vi "play-general-scan-with-autoID.vi"() -> ()   [LabVIEW 2017]
uses:
  <vilib>/addons/Control Design/_Model Construction/Model Typedefs.llb/CD State Space Model (MIMO).ctl
  <vilib>/addons/Control Design/_Model Construction/Model Typedefs.llb/CD General Elements.ctl
  fpga_VIs/fpga_subVIs_ssxy/fixed-point-ss/typeDefs/FXPControlParams-ss-xy.ctl
  controls/z-axis-params_v4_prescan.ctl
  controls/TF-params.ctl
  controls/scan_input_meta_data.ctl
  controls/scan-mode-CTL.ctl
  fpga_VIs/controls/supervisor-params.ctl
  fpga_VIs/controls/fpga-scan-status.ctl
  controls/boolean_info.ctl
  controls/auto_id_result.ctl
  subVIs/auto-sys-id/controls/SOS_frf_data.ctl
  fpga_interface_lib/fpga_interface_types/cs-scan-inputs-TYPE.ctl
  <vilib>/userdefined/High Color/nirio_resource_hc.ctl
  controls/rasterMetaData_asCS.ctl
  <vilib>/FPGAPlugInAG/cRIO-9082/niLvFpga_Open_cRIO-9082.vi
  <vilib>/rvi/interface/common/dynamic/niFpgaDynamicAddResources.vi
  <vilib>/FPGAPlugInAG/Dynamic/niLvFpga_Reset_Dynamic.vi
  <vilib>/Utility/error.llb/Error Cluster From Error Code.vi
  <vilib>/rvi/errors/niLvFpgaAdjustHostInterfaceError.vi
  <vilib>/FPGAPlugInAG/Dynamic/niLvFpga_Run_Dynamic.vi
  fpga_interface_lib/acquire_FXP_16-5_FIFO_2.vi
  <vilib>/RVI Host/nirviSupport.llb/nirviErrorClusterFromErrorCode.vi
  <vilib>/FPGAPlugInAG/Dynamic/niLvFpga_Close_Dynamic.vi
  <vilib>/rvi/interface/nirviOpenFPGA/nirviOpenFPGA.xnode
  FPGA Bitfiles/afmimagingcontro_FPGATargetSPARTA_cs-scanningv5ssx.lvbitx
  <vilib>/rvi/interface/nirviMethod/nirviMethod.xnode
  <vilib>/rvi/interface/nirviReadWriteControl/nirviReadWriteControl.xnode
  <vilib>/rvi/interface/nirviCloseFPGA/nirviCloseFPGA.xnode
  <vilib>/rvi/interface/Simulation/niFpgaSimulationCallBeginRW.vi
  NiFpgaLv.dll
  fpga_interface_lib/fpga_interface.lvlib
  <vilib>/addons/_JKI.lib/Serialization/JSON/JKI JSON Serialization.lvlib
  <vilib>/rvi/interface/nirviMethod/StockFPGA_InlinedMethodWaitForSingleIRQ.vi
  <vilib>/FPGAPlugInAG/Dynamic/niLvFpga_WaitOnIrq_Dynamic.vi
  <vilib>/FPGAPlugInAG/Dynamic/niLvFpga_AcknowledgeIrq_Dynamic.vi
  <vilib>/addons/Control Design/_Model Construction/NI_LinSys_Model Typedefs.lvlib
panel:
  out "Array 3":T1(array[cluster])
  out "current-acquisition":i32
  out "state0-count":u64
  out "output cluster":T2={"xy_settled_samples_threshold"=15, "xy_error_threshold"=0.01, "zup_err_threshold"=0.10000228881835938, "prescan_samples"=5000, "TOL"=0.3, "collect_all"=TRUE, "numEntities"=0} {"TOL" format="%#_13g"}
  out "current-state":u8
  in  "Alert-on-Finish":bool
  out "state times":dbl[](array[numeric])
  out "ControlMatrices":T3
  in  "Tab Control":T4(tab)
  in  "Array 4":path[](array[path])
  in  "z_axis_params":T5={"z_u_max"=2.0, "setpoint_scan"=-0.3000030517578125, "Ki_scan"=0.07, "uz_safe"=0.2998046875, "Kiz_down"=0.045, "setpoint_up"=-0.8000030517578125, "do_Dz"=TRUE, "PID_while_xy_move"=FALSE, "TF_params"={"TF_order"=2, "Num"=[1.0, -1.9962076, 0.9990926, 0.0, 0.0, 0.0, 0.0, 0.0, 0.0], "Den"=[1.0, -1.9961313, 0.9990842, 0.0, 0.0, 0.0, 0.0, 0.0, 0.0]}, "KI_slope"=1.0, "enable_KI_sched"=FALSE, "KI_min"=0.0099945068359375, "KI_max"=0.1999969482421875} {"Kiz_down" format="%#_13g"; "Ki_scan" min=0 max=0.4 step=0.0025; "z_u_max" format="%#_13g"}
  in  "overwrite":bool
  in  "note-blob":string
  in  "state-machine-params":T2={"xy_settled_samples_threshold"=20, "xy_error_threshold"=0.01, "zup_err_threshold"=0.05100059509277344, "prescan_samples"=0, "TOL"=0.0259, "collect_all"=TRUE, "numEntities"=0} {"TOL" format="%#_13g"}
  in  "trigger-0":bool
  in  "STOP":bool
  out "CS Time":dbl
  in  "collect-0":bool
  in  "Continue":bool
  out "output-data-paths":path[](array[path])
  in  "file path (use dialog)":path=path "C:/Users/arnold/Documents/afm-cs/labview/first_res_fit-5-9-2019-sicon.json"
  in  "xy-gain-mult":dbl=1.0 min=0.0 max=1.0 step=1.0 format="%#_13g"
  in  "Load-Dinv":bool=TRUE
  in  "Swept-Sines-Control-Settings":cluster{"u-max":sgl, "offset":sgl, "Ki":sgl}={"u-max"=1.0, "offset"=0.1, "Ki"=0.0}
  in  "SS-amp":dbl=0.12 format="%#_13g"
  out "Bode amplitude":cluster{"W":dbl[], "Magnitude":dbl[]}[](graph) caption="Magnitude Graph"
  out "Channel 1":cluster{"W":dbl[], "Magnitude":dbl[]}[](graph) caption="Magnitude Graph"
  out "value":T7
  in  "Abort-swept-sines":bool
  in  "control_data_path":path=path "Z:/afm-cs/step-exps/LinControls-choose-zeta_5micron.json"
  in  "umax-xy":dbl=5.0 format="%#_13g"
  out "Gdrift-inv-xdir":T9 {"Transport Delay" format="%.2f"; "D" format="%#.5g"; "C" format="%#.5g"; "B" format="%#.5g"; "A" format="%#.5g"; "properties"."Sampling Time" format="%#.6p"; "properties"."Output Delays" format="%.4f"; "properties"."Input Delays" format="%.4f"}
  out "ControlParamsLin-ss":T11={"umax"=3.0, "Ns_obs/cntrl"=0, "ref_f_VEC"=[0.0, 0.0], "du_max"=0.0, "Nbar"=0.0, "Nhyst"=0, "Nsat"=0, "Ndrift+1"=0, "Ki-y"=0.01}
  in  "Ki-y":sgl=0.01
  out "scan-status":T12
  out "error out 2":errorcluster
  out "scan_meta":T14
  out "Kiscan-effective":dbl
  out "Kidown-effective":dbl
  out "K":dbl
  out "error out":errorcluster
  out "output-meta-data-path":path
  # "C:\\Users\\arnold\\Documents\\afm-cs\\labview\\first_res_fit-4-19-2019-sicon.json"
  # "make this come from input csv!"
  # "For the y-axis only, shouldnt ever really\nneed to change"
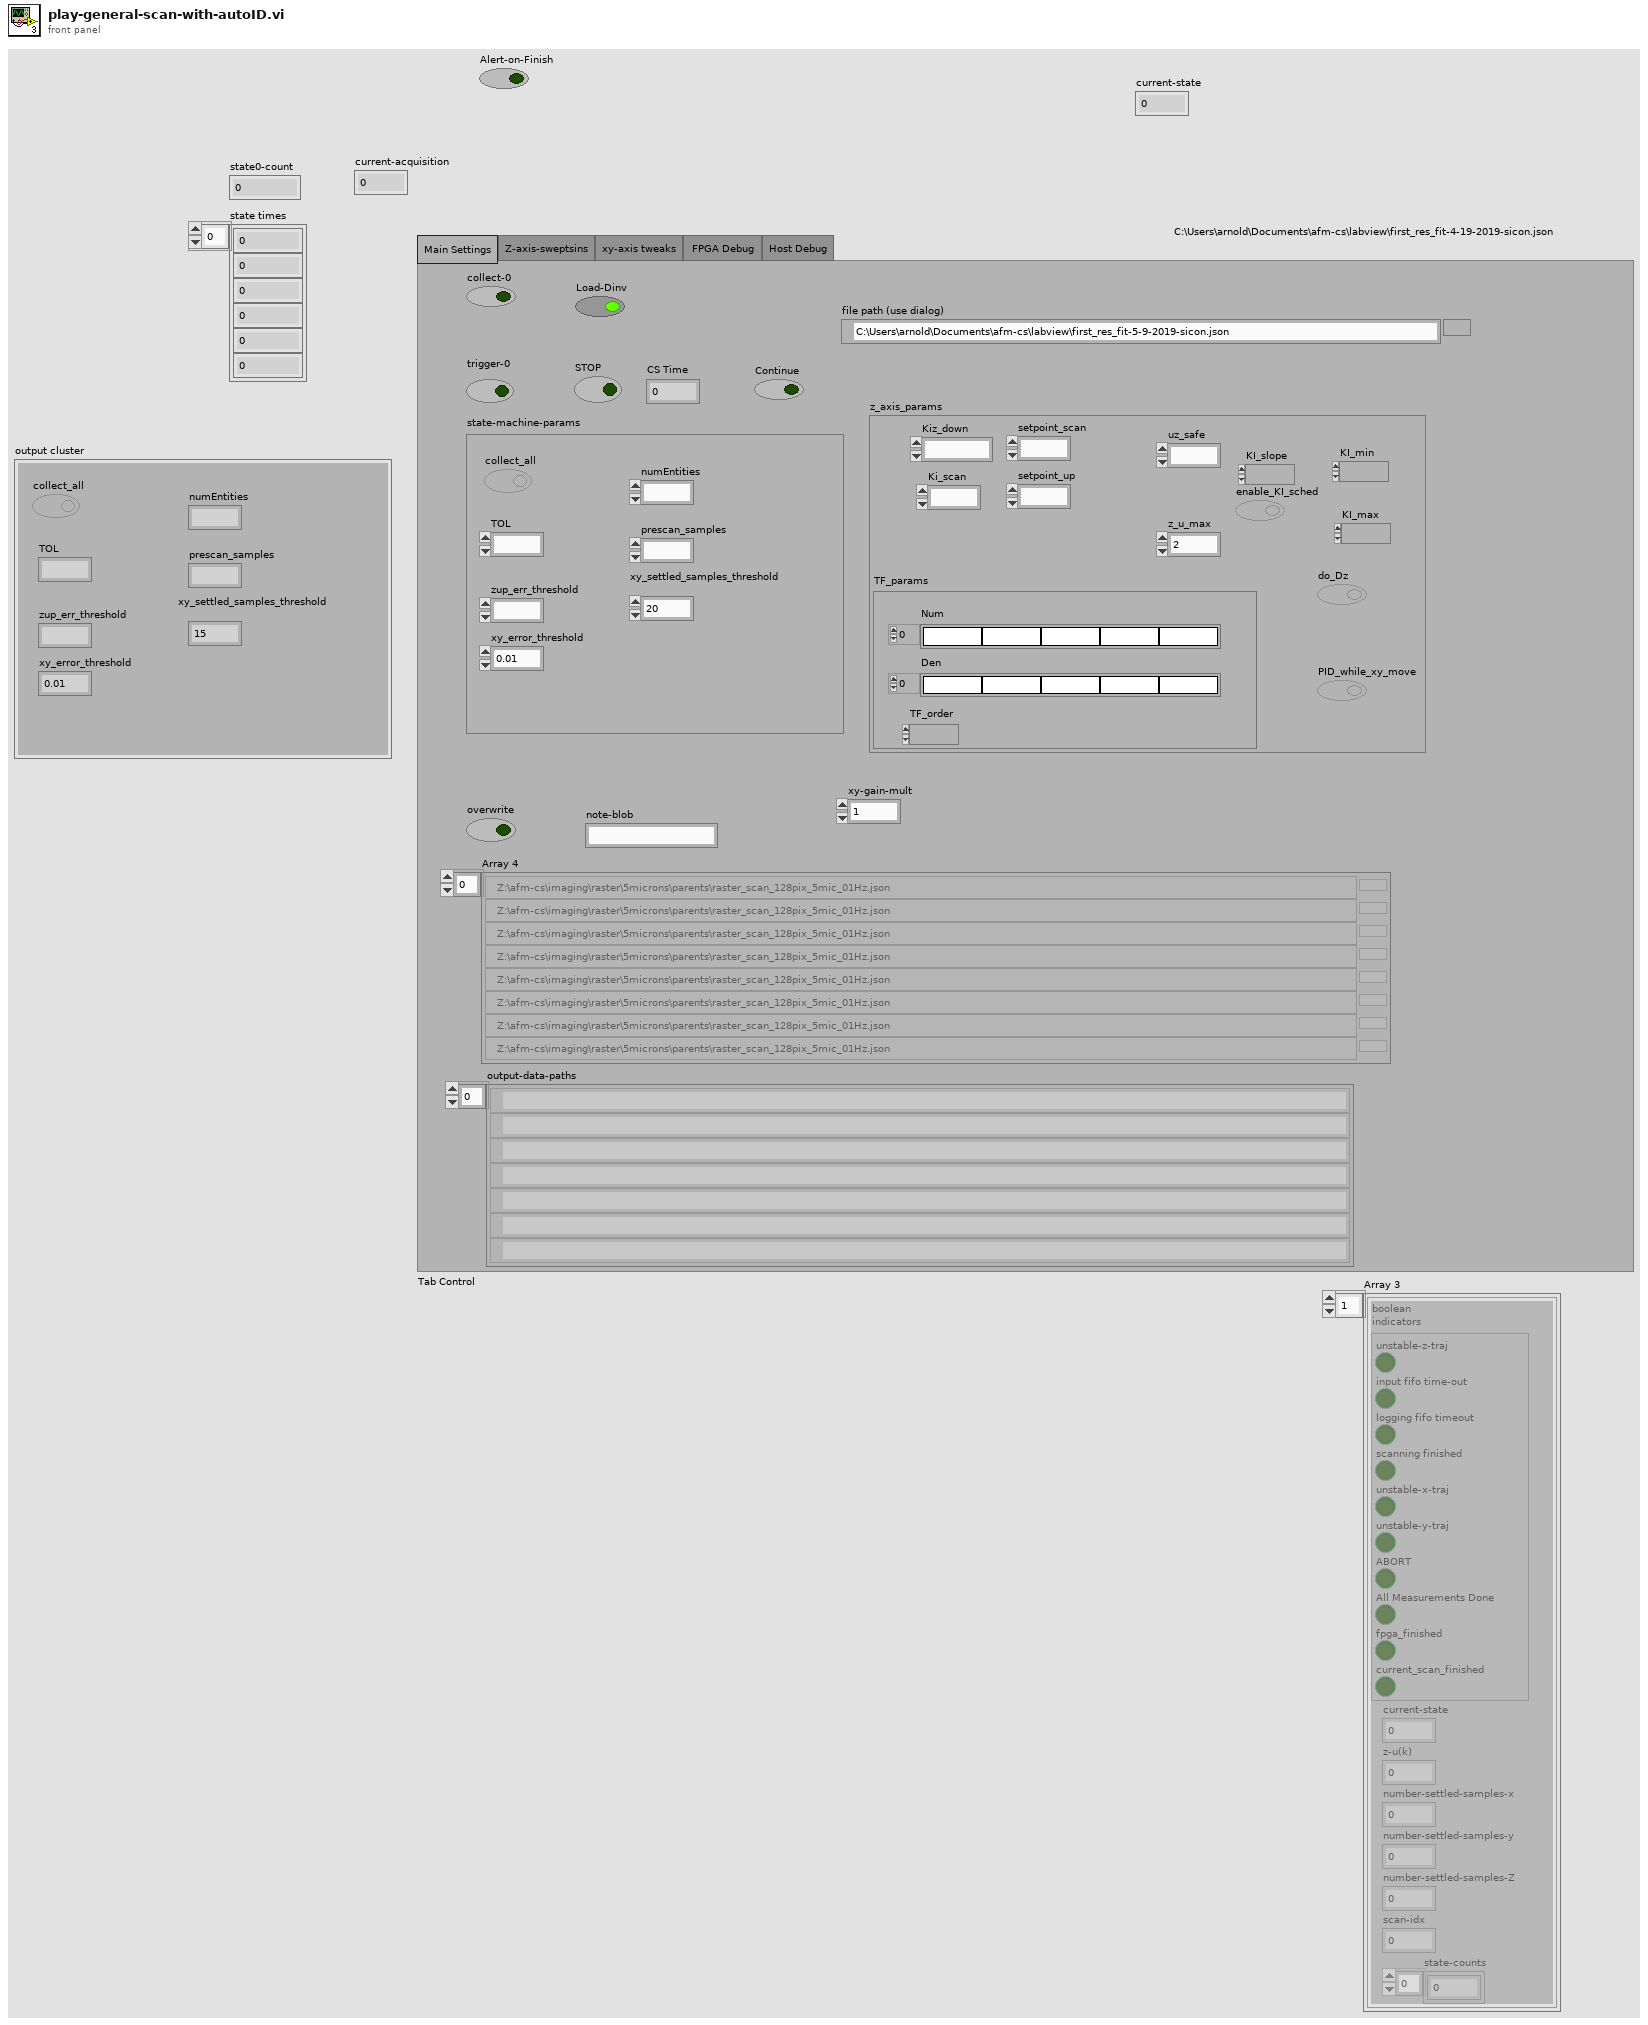
[diagram p1: front panel]
types:
  T1 = cluster{"boolean \nindicators":cluster{"unstable-z-traj":bool, "input fifo time-out":bool, "logging fifo timeout":bool, "scanning finished":bool, "unstable-x-traj":bool, "unstable-y-traj":bool, "ABORT":bool, "All Measurements Done":bool, "fpga_finished":bool, "current_scan_finished":bool}, "current-state":u8, "z-u(k)":sgl, "number-settled-samples-x":i16, "number-settled-samples-y":i16, "number-settled-samples-Z":i16, "scan-idx":i16, "state-counts":u64[]}[]
  T2 = typedef "supervisor-params.ctl" = cluster{"xy_settled_samples_threshold":i16, "xy_error_threshold":sgl, "zup_err_threshold":fxp<+,24,5>, "prescan_samples":i16, "TOL":sgl, "collect_all":bool, "numEntities":i16}
  T3 = cluster{"Az":fxp<+/-,32,4>[][], "Bz":dbl[][], "Lz":dbl[][], "Kz":dbl[][], "NxNu":dbl[][]}
  T4 = enum32{"Main Settings", "Z-axis-sweptsins", "xy-axis tweaks", "FPGA Debug ", "Host Debug"}
  T5 = typedef "z-axis-params_v4_prescan.ctl" = cluster{"z_u_max":sgl, "setpoint_scan":fxp<+/-,32,16>, "Ki_scan":sgl, "uz_safe":fxp<+/-,16,5>, "Kiz_down":sgl, "setpoint_up":fxp<+/-,32,16>, "do_Dz":bool, "PID_while_xy_move":bool, "TF_params":T6, "KI_slope":fxp<+/-,32,16>, "enable_KI_sched":bool, "KI_min":fxp<+/-,32,16>, "KI_max":fxp<+/-,32,16>}
  T6 = typedef "TF-params.ctl" = cluster{"TF_order":i16, "Num":sgl[], "Den":sgl[]}
  T7 = typedef "auto_id_result.ctl" = cluster{"Dinv_Num":dbl[], "SOS_frf_data":T8, "Dinv_den":dbl[], "K":dbl}
  T8 = typedef "SOS_frf_data.ctl" = cluster{"omegas":dbl[], "resp_real":dbl[], "resp_imag":dbl[], "theta0":dbl[]}
  T9 = typedef "NI_LinSys_Model Typedefs.lvlib/CD State Space Model (MIMO).ctl" = cluster{"properties":T10, "A":dbl[][], "B":dbl[][], "C":dbl[][], "D":dbl[][], "StateNames":string[], "Transport Delay":dbl[][]}
  T10 = typedef "NI_LinSys_Model Typedefs.lvlib/CD General Elements.ctl" = cluster{"Model name":string, "Input names":string[], "Output names":string[], "Input Delays":dbl[], "Output Delays":dbl[], "Sampling Time":dbl, "Notes":string}
  T11 = typedef "FXPControlParams-ss-xy.ctl" = cluster{"umax":fxp<+/-,18,5>, "Ns_obs/cntrl":u8, "ref_f_VEC":fxp<+/-,32,5>[], "du_max":fxp<+/-,18,5>, "Nbar":fxp<+/-,32,5>, "Nhyst":u8, "Nsat":u8, "Ndrift+1":u8, "Ki-y":sgl}
  T12 = typedef "fpga-scan-status.ctl" = cluster{"boolean \nindicators":T13, "current-state":u8, "z-u(k)":sgl, "number-settled-samples-x":i16, "number-settled-samples-y":i16, "number-settled-samples-Z":i16, "scan-idx":i16, "state-counts":u64[]}
  T13 = typedef "boolean_info.ctl" = cluster{"unstable-z-traj":bool, "input fifo time-out":bool, "logging fifo timeout":bool, "scanning finished":bool, "unstable-x-traj":bool, "unstable-y-traj":bool, "ABORT":bool, "All Measurements Done":bool, "fpga_finished":bool, "current_scan_finished":bool}
  T14 = typedef "scan_input_meta_data.ctl" = cluster{"npix":i64, "raster_freq":dbl, "width":dbl, "points_per_line":i64, "points_per_period":i64, "total_num_points":i64, "scan_type":T15, "number_of_scans":i64, "actual_sub_samble_perc":dbl, "mu_length":dbl, "tip_velocity":dbl, "pix_idx":i32[], "overscan_samples":i16, "pre_scan_samples":i16}
  T15 = typedef "scan-mode-CTL.ctl" = enum16{"raster", "CS"}
  T16 = enum16{"open", "replace", "create", "open or create", "replace or create", "replace or create with confirmation"}
  T17 = typedef "fpga_interface.lvlib/cs-scan-inputs-TYPE.ctl" = refnum<k20>
  T18 = typedef "rasterMetaData_asCS.ctl" = cluster{"Ki_xy":dbl, "number_of_lines":i32, "Ki_derate":sgl, "ze_sched_thresh":sgl, "scan_meta":T14, "z_axis_params":T5, "state_counts":dbl[], "state_machine_params":T2, "input_data_path":path, "output_data_path":path, "xy_control_path":path}
  T19 = typedef "nirio_resource_hc.ctl" = tag
  T20 = typedef "ObserverMatrices.ctl" = cluster{"Az":fxp<+/-,32,4>[][], "Bz":dbl[][], "Lz":dbl[][], "Kz":dbl[][], "NxNu":dbl[][]}
  T21 = cluster{"boolean \nindicators":cluster{"unstable-z-traj":bool, "input fifo time-out":bool, "logging fifo timeout":bool, "scanning finished":bool, "unstable-x-traj":bool, "unstable-y-traj":bool, "ABORT":bool, "All Measurements Done":bool, "fpga_finished":bool, "current_scan_finished":bool}, "current-state":u8, "z-u(k)":sgl, "number-settled-samples-x":i16, "number-settled-samples-y":i16, "number-settled-samples-Z":i16, "scan-idx":i16, "state-counts":u64[]}
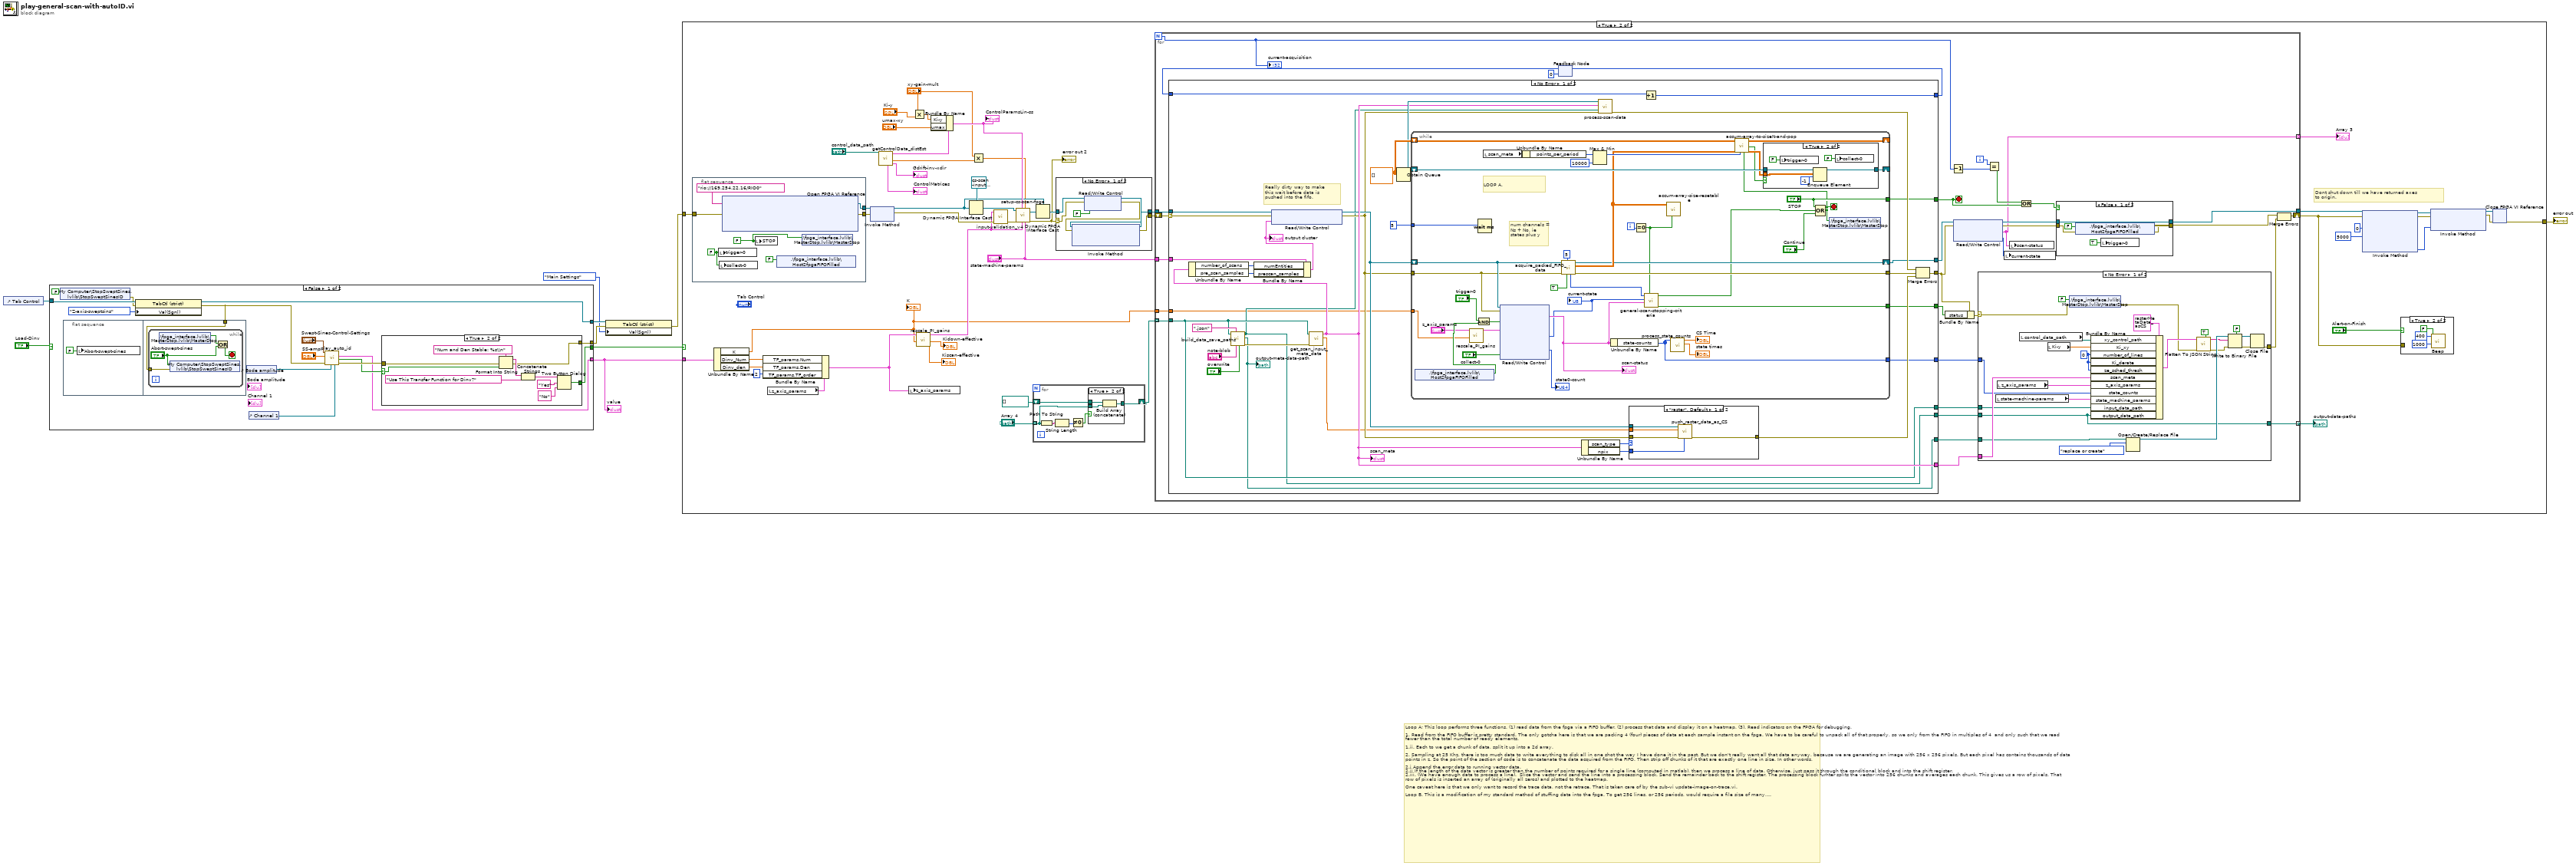
[diagram p0: block diagram]
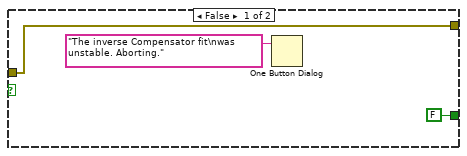
[diagram p2: hidden frame]
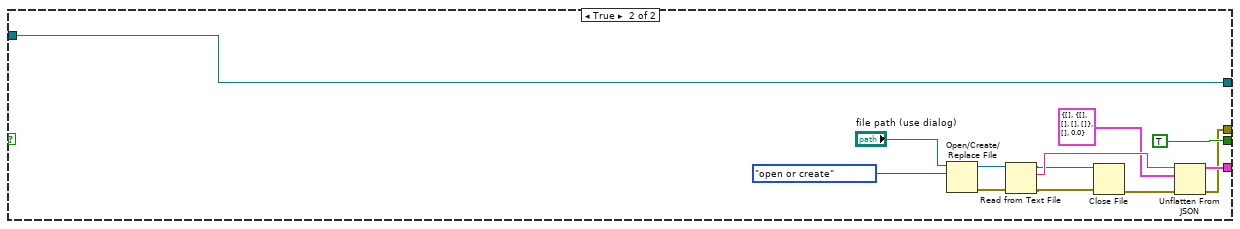
[diagram p3: hidden frame]
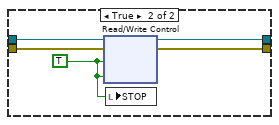
[diagram p7: hidden frame]
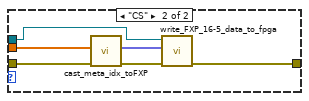
[diagram p9: hidden frame]
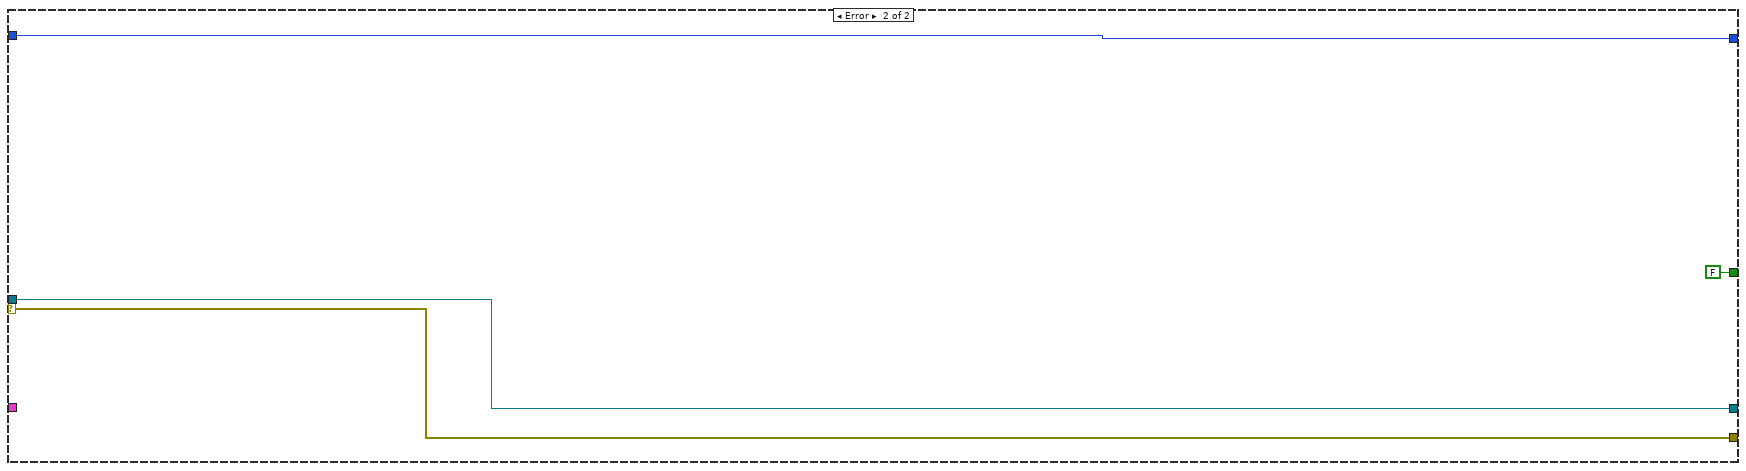
[diagram p11: hidden frame]
diagram:
  # "Loop A; This loop performs three functions. (1) read data from the fpga via a FIFO buffer. (2) process that data and display it on a heatmap. (3). Read indicators on the FPGA for debugging.\n\n1. Read from the FIFO buffer is pretty standard. The only gotcha here is that we are packing 4 (four) pieces of data at each sample instant on the fpga. We have to be careful to unpack all of that properly, so we only from the FIFO in multiples of 4  and only such that we read fewer than the total number of ready elements. \n\n1.ii. Each to we get a chunk of data, split it up into a 2d array. \n\n2. Sampling at 25 Khz, there is too much data to write everything to disk all in one shot the way I have done it in the past. But we don't really want all that data anyway, because we are generating an image with 256 x 256 pixels. But each pixel has contains thousands of data points in z. So the point of the section of code is to concatenate the data acquired from the FIFO. Then strip off chunks of it that are exactly one line in size. In other words,\n\n2.i Append the error data to running vector data.\n2.ii If the length of the data vector is greater than the number of points required for a single line (computed in matlab), then we process a line of data. Otherwise, just pass it through the conditional block and into the shift register. \n2.iii. (We have enough data to process a line).  Slice the vector and send the line into a processing block. Send the remainder back to the shift register. The processing block furhter splits the vector into 256 chunks and averages each chunk. This gives us a row of pixels. That row of pixels is inserted an array of (originally all zeros) and plotted to the heatmap.\n\nOne caveat here is that we only want to record the trace data, not the retrace. That is taken care of by the sub-vi update-image-on-trace.vi.\n\nLoop B. This is a modification of my standard method of stuffing data into the fpga. To get 256 lines, or 256 periods, would require a file size of many, many gigibtyes. SO the point here is to only use a single period of the triangle wave and corresponding ramp signal. Everytime we exauhst that data, re-cycle the same data and keep pumping it back in. The one tricky part here is that we have to be careful to shift the original ramp data up by the appropriate amount. We also have to take special care because of how the data is packed from matlab. [x(1), y(1), x(2), y(2)...].\n\nThe first iteration of the loop, we don't push any data in. All we do is get the number of empty elements.\n\nB.1 Each iteration, strip off ' empty elements ' elements from the array and send them to FIFO. \nB.2.i Is the remaining array empty?\nB.2.ii Grab the very last element. We need this"
  n1 = control-ref of="Tab Control"() -> (w6:refnum<vi>)
  n2 = case shown="False" "Load-Dinv" {
    tunnel: [w18 w47] -> w9
    tunnel: [w20 TRUE] -> w8
    tunnel: [w19 w45] -> w4
    tunnel: w6 -> [w14 w44]
    tunnel: [w13 w44] -> w5
    frame False {
      n3 = shared-variable "My Computer\\StopSweptSines.lvlib\\StopSweptSinesID"(FALSE ("StopSweptSinesID")) -> (error out=w12:errorcluster)  [unwired: 1 in]
      n4 = flat-sequence {
        tunnel: w10 -> [w26]
        frame #0 {
          n5 = local write "Abort-swept-sines"(FALSE ("Abort-swept-sines")) -> ()
        }
        frame #1 {
          n6 = while {
            tunnel: w26 -> [w30]
            stop <- w28 stop-if-true
            n7 = shared-variable ".\\fpga_interface.lvlib\\MasterStop.lvlib\\MasterStop"() -> (w29:bool)  [unwired: 1 in, 1 out]
            n8 = shared-variable "My Computer\\StopSweptSines.lvlib\\StopSweptSinesID"("Abort-swept-sines", error in=w30) -> ()  [unwired: 1 out]
            n9 = Or(x=w29, y="Abort-swept-sines") -> (x .or. y?=w28:bool)
          }
        }
      }
      n10 = property class="TabCtl (strict)"(reference=w14, error in=w12, "Val(Sgnl)"=T4."Z-axis-sweptsins" ("Value (Signaling)")) -> (reference out=w13:refnum<vi>, error out=w10:errorcluster)
      n11 = control-ref of="Bode amplitude"() -> (w17:refnum<vi>)
      n12 = control-ref of="Channel 1"() -> (w16:refnum<vi>)
      n13 = call "play_auto_id.vi"("time-series-in"=w16, "Bode amplitude_in"=w17, "error in"=w10, "Amplitude"="SS-amp", "Swept-Sines-Control-Settings"="Swept-Sines-Control-Settings") -> ("error out"=w24:errorcluster, "Is-Totally-Stable"=w23:bool, "auto_id_result"=w18:T7)  [unwired: 4 in]
      n14 = case shown="True" w23 {
        selector: w23 -> [_ w35]
        tunnel: [FALSE ("T button?") w43] -> w20
        tunnel: [w31 w37] -> w19
        tunnel: w24 -> [w31 w36]
        frame False {
          n15 = One Button Dialog(message="The inverse Compensator fit\nwas unstable. Aborting.") -> ()  [unwired: 1 in, 1 out]
        }
        frame True {
          n16 = Format Into String(format string="Num and Den Stable: %s\\n" ("initial string"), error in=w36, w35) -> (resulting string=w39:string, error out=w37:errorcluster)  [unwired: 1 in]
          n17 = Concatenate Strings(w39, "Use This Transfer Function for Dinv?" ("message")) -> (w38:string)
          n18 = Two Button Dialog(message=w38, 1:"No" ("F button name (\"Cancel\")"), 2:"Yes" ("T button name (\"OK\")")) -> (T button?=w43:bool)
        }
      }
    }
    frame True {
      n19 = Open/Create/Replace File(file path (use dialog)="file path (use dialog)", operation (0:open)=T16."open or create") -> (refnum out=w52:refnum<file>, error out=w51:errorcluster)  [unwired: 4 in, 1 out]
      n20 = Read from Text File(file (use dialog)=w52, error in=w51) -> (refnum out=w53:refnum<file>, text=w55:string, error out=w54:errorcluster)  [unwired: 2 in, 1 out]
      n21 = Close File(refnum=w53, error in=w54) -> (error out=w56:errorcluster)  [unwired: 1 out]
      n22 = Unflatten From JSON(JSON string=w55, type and defaults=T7 {"Dinv_Num"=[], "SOS_frf_data"={"omegas"=[], "resp_real"=[], "resp_imag"=[], "theta0"=[]}, "Dinv_den"=[], "K"=0.0} ("auto_id_result 2"), error in (no error)=w56) -> (value=w47:T7, error out=w45:errorcluster)  [unwired: 4 in]
    }
  }
  "value" <- w9
  n23 = property class="TabCtl (strict)"(reference=w5, error in=w4, "Val(Sgnl)"=T4."Main Settings" ("Value (Signaling)")) -> (error out=w3:errorcluster)  [unwired: 1 out]
  n24 = case shown="True" w8 {
    tunnel: w9 -> [_ w63]
    tunnel: w3 -> [w57 w59]
    tunnel: [w57 w58] -> w7
    frame False {
    }
    frame True {
      # "Dont shut down till we have returned axes\nto origin."
      n25 = flat-sequence {
        tunnel: [w298] -> w108
        tunnel: [w297] -> w107
        tunnel: w59 -> [w292]
        frame #0 {
          w293 = FALSE ("trigger-0")
          w295 = FALSE
          n26 = local write "trigger-0"(w293) -> ()
          n27 = local write "collect-0"(w293) -> ()
          n28 = xnode "Open FPGA VI Reference"("error in"=w292, "resource name"=T19 "rio://169.254.22.16/RIO0") -> ("FPGA VI Reference Out"=w298:refnum<k20>, "error out"=w297:errorcluster)
          n29 = local write "STOP"(w295) -> ()
          n30 = shared-variable ".\\fpga_interface.lvlib\\Host2fpgaFIFOFilled"(FALSE ("Host2fpgaFIFOFilled")) -> ()  [unwired: 1 in, 1 out]
          n31 = shared-variable ".\\fpga_interface.lvlib\\MasterStop.lvlib\\MasterStop"(w295) -> ()  [unwired: 1 in, 1 out]
        }
      }
      n32 = Unbundle By Name(w63) -> ("K"=w60:dbl, "Dinv_Num"=w66:dbl[], "Dinv_den"=w65:dbl[])
      "K" <- w60
      n33 = local read "z_axis_params"() -> (w61:T5)
      n34 = Bundle By Name(cluster=w61, "TF_params.Num"=w66, "TF_params.Den"=w65, "TF_params.TF_order"=i16 2) -> (w62:T5)
      n35 = xnode "Invoke Method"("FPGA VI Reference In"=w108, "error in"=w107) -> ("FPGA VI Reference Out"=w80:refnum<k20>, "error out"=w86:errorcluster)
      n36 = call "getControlData_distEst.vi"("system data path"="control_data_path") -> ("Gdrift"=→"Gdrift-inv-xdir":T9, "AllMatrix"=w72:dbl[], "ControlParams"=w105:T11, "ControlMatrices"=→"ControlMatrices":T20)  [unwired: 7 in]
      n37 = local write "z_axis_params"(w62) -> ()
      n38 = Multiply(x="xy-gain-mult", y="Ki-y") -> (x*y=w70:dbl)
      n39 = call "rescale_PI_gains.vi"("Dinv-k"=w60, "z-axis-params-in"=w62) -> ("Kiscan-effective"=→"Kiscan-effective":dbl, "Kidown-effective"=→"Kidown-effective":dbl, "z-axis-params-out"=w75:T5)  [unwired: 7 in]
      n40 = Bundle By Name(cluster=w105, "Ki-y"=w70, "umax"="umax-xy") -> (w87:T11)
      "ControlParamsLin-ss" <- w87
      n41 = Dynamic FPGA Interface Cast(Session In=T17 refnum ("FPGA Interface in"), Type=w80) -> (Session Out=w89:T17)
      n42 = Multiply(x="xy-gain-mult", y=w72) -> (x*y=w71:dbl[])
      n43 = call "input-validation_v4.vi"("error constant"=w86, "z_axis_params"=w75) -> ("error out"=w82:errorcluster)  [unwired: 9 in]
      n44 = call "setup-cs-scan-fpga.vi"("state-machine-params"="state-machine-params", "Control-matrices"=w71, "z_axis_params"=w75, "ControlParamsLin-ss"=w87, "error in"=w82, "FPGA Interface in"=w89) -> ("error out"=w81:errorcluster, "FPGA Interface out"=w84:T17)  [unwired: 4 in]
      "error out 2" <- w81
      n45 = for {
        tunnel: "Array 4" -> [w109] mode=indexing
        shift-right: [w112] -> w76
        shift-left: path[] [] -> [w113]
        n46 = Path To String(path=w109) -> (string=w114:string)
        n47 = String Length(string=w114) -> (length=w110:i32)
        n48 = Not Equal To 0?(x=w110) -> (x != 0?=w111:bool)
        n49 = case shown="True" w111 {
          tunnel: w113 -> [w115 w117]
          tunnel: [w115 w118] -> w112
          tunnel: w109 -> [_ w116]
          frame False {
          }
          frame True {
            n50 = Build Array (concatenate)(w117, w116) -> (w118:path[])
          }
        }
      }
      n51 = Dynamic FPGA Interface Cast(Session In=w80, Type=w84) -> (Session Out=w85:refnum<k20>)
      n52 = case shown="No Error" w81 {
        selector: w81 -> [w285 w290]
        tunnel: w85 -> [w286 w291]
        tunnel: [w289 w290] -> w101
        tunnel: [w288 w291] -> w100
        frame No Error {
          n53 = xnode "Read/Write Control"("FPGA VI Reference In"=w286, "error in"=w285, "trigger-0"=FALSE) -> ("FPGA VI Reference Out"=w284:refnum<k20>, "error out"=w287:errorcluster)
          n54 = xnode "Invoke Method"("FPGA VI Reference In"=w284, "error in"=w287) -> ("FPGA VI Reference Out"=w288:refnum<k20>, "error out"=w289:errorcluster)  [unwired: 1 in]
        }
        frame Error {
        }
      }
      n55 = for {
        N -> [w133]
        shift-right: [w142] -> w91
        shift-left: w101 -> [w151]
        tunnel: w100 -> [w150]
        tunnel: [w143] -> w90
        tunnel: "state-machine-params" -> [w137]
        tunnel: w76 -> [w134] mode=indexing
        tunnel: [w129] -> w79 mode=indexing
        tunnel: [w126] -> w78 mode=indexing
        tunnel: w60 -> [w122]
        i -> [w138]
        stop <- w147 stop-if-true
        n56 = feedback #1(i16 0) -> (w131:i16)
        n57 = case shown="No Error" w151 {
          selector: w151 -> [w204 w280]
          tunnel: [w219 w280] -> w125
          tunnel: [w210 w281] -> w149
          tunnel: w150 -> [w205 w281]
          tunnel: [w200 _] -> w153
          tunnel: [w212 _] -> w152
          tunnel: [w211 FALSE ("STOP")] -> w147
          tunnel: w137 -> [w193 _]
          tunnel: w134 -> [w199 _]
          tunnel: [w199 _] -> w136
          tunnel: [w198 _] -> w135
          tunnel: [w195 w279] -> w132
          tunnel: w131 -> [w194 w279]
          tunnel: [w192 _] -> w127
          tunnel: [w191 _] -> w123
          tunnel: w122 -> [w190 _]
          frame No Error {
            w217 = dbl[][] []
            # "Really dirty way to make\nthis wait before data is\npushed into the fifo."
            n58 = call "build_data_save_paths.vi"("overwrite"="overwrite", "note-blob"="note-blob", "meta-file-ext"=".json" ("replace string (\"\")"), "input-file"=w199) -> ("error IO"=w209:errorcluster, "output-meta-data-path"=w198:path, "output-data-path"=w192:path)  [unwired: 4 in, 1 out]
            "output-meta-data-path" <- w198
            n59 = call "get_scan_input_meta_data.vi"("error in"=w209, "Path"=w199) -> ("fpga_input"=w189:dbl[], "meta_data"=w200:T14)  [unwired: 7 in, 1 out]
            "scan_meta" <- w200
            n60 = Unbundle By Name(w200) -> ("number_of_scans"=w202:i64, "pre_scan_samples"=w203:i16)
            n61 = Bundle By Name(cluster=w193, "numEntities"=w202, "prescan_samples"=w203) -> (w201:T2)
            "output cluster" <- w201
            n62 = xnode "Read/Write Control"("FPGA VI Reference In"=w205, "error in"=w204, "state-machine-params"=w201) -> ("FPGA VI Reference Out"=w197:refnum<k20>, "error out"=w196:errorcluster)
            n63 = Obtain Queue(element data type=w217) -> (queue out=w215:refnum<queue>)  [unwired: 4 in, 2 out]
            n64 = while {
              tunnel: 5 -> [w271]
              tunnel: [w267] -> w220
              shift-right: [w270] -> _
              shift-left: w215 -> [w269]
              tunnel: w196 -> [w249]
              tunnel: [w255] -> w212
              shift-right: [w263] -> _
              shift-left: w217 -> [w262]
              tunnel: ["STOP"] -> w211
              shift-right: [w252] -> w210
              shift-left: w197 -> [w250]
              tunnel: [w237] -> w191
              tunnel: w190 -> [w233]
              i -> [w253]
              stop <- w236 stop-if-true
              # "LOOP A."
              # "num channels = Ns + No, ie states plus y"
              n65 = shared-variable ".\\fpga_interface.lvlib\\Host2fpgaFIFOFilled"() -> (w245:bool)  [unwired: 1 in, 1 out]
              n66 = call "rescale_PI_gains.vi"("Dinv-k"=w233, "z-axis-params-in"="z_axis_params") -> ("z-axis-params-out"=w235:T5)  [unwired: 7 in, 2 out]
              n67 = And(x="trigger-0", y=w245) -> (x .and. y?=w248:bool)
              n68 = Wait (ms)(milliseconds to wait=w271) -> ()  [unwired: 1 out]
              n69 = local read "scan_meta"() -> (w259:T14)
              n70 = xnode "Read/Write Control"("FPGA VI Reference In"=w250, "error in"=w249, "trigger-0"=w248, "z_axis_params"=w235, "collect-0"="collect-0") -> ("scan-status"=w243:T21, "current-state"=w242:u8, "state0-count"=→"state0-count":u64)  [unwired: 3 out]
              "scan-status" <- w243
              "current-state" <- w242
              n71 = Unbundle By Name(w259) -> ("points_per_period"=w258:i64)
              n72 = call-poly "acquire_packed_FIFO_data.vi"("Run once?"=TRUE, "numChannels"=u32 5 ("y"), "error in"=w249, "FPGA Interface(in)"=w250) -> ("error out"=w267:errorcluster, "2D Data Out"=w254:dbl[][], "FPGA VI Reference Out"=w252:refnum<k20>, "Elements Remaining"=w241:u32)  [unwired: 3 in, 1 out]
              n73 = Max & Min(x=w258, y=i64 10000) -> (max(x,y)=w256:i64)  [unwired: 1 out]
              n74 = Unbundle By Name(w243) -> ("state-counts"=w255:u64[])
              n75 = Equal To 0?(x=w253) -> (x = 0?=w240:bool)
              n76 = call "general-scan-stopping-criteria.vi"("reset"=w240, "scan-status"=w243, "current-state"=w242, "FIFO-elementas-left"=w241) -> ("FIFO timeout"=w237:bool, "Finish"=w239:bool)  [unwired: 6 in]
              n77 = call "accum-array-size-resetable.vi"("reset"=w240, "array"=w254) -> ()  [unwired: 9 in, 1 out]
              n78 = call "process_state_counts.vi"("state-counts"=w255) -> ("State_times"=→"state times":dbl[], "Cs_time"=→"CS Time":dbl)  [unwired: 9 in]
              n79 = Compound Arithmetic op=OR("STOP", w239, "Continue") -> (w236:bool)
              n80 = call "accum-array-to-sizeN-and-pop.vi"("flush"=w236, "Nsize"=w256, "new-data-in"=w254, "old-data-in"=w262) -> ("popped-data"=w261:dbl[][], "new-data-ready"=w260:bool, "old-data-out"=w263:dbl[][])  [unwired: 5 in]
              n81 = case shown="True" w260 {
                tunnel: w269 -> [w272 w278]
                tunnel: w261 -> [_ w276]
                tunnel: [w272 w275] -> w270
                frame False {
                }
                frame True {
                  n82 = local write "trigger-0"(FALSE ("trigger-0")) -> ()
                  n83 = Enqueue Element(queue=w278, element=w276, timeout in ms (-1)=-1) -> (queue out=w275:refnum<queue>)  [unwired: 1 in, 2 out]
                  n84 = local write "collect-0"(FALSE ("collect-0")) -> ()
                }
              }
              n85 = shared-variable ".\\fpga_interface.lvlib\\MasterStop.lvlib\\MasterStop"(w236) -> ()  [unwired: 1 in, 1 out]
            }
            n86 = Unbundle By Name(w200) -> ("scan_type"=w213:T15, "npix"=w216:i64)
            n87 = call "process-scan-data.vi"("error in"=w196, "output-data-path"=w192, "scan_meta"=w200, "queue in"=w215) -> ("error out"=w214:errorcluster)  [unwired: 7 in]
            n88 = case shown="\"raster\", Default" w213 {
              tunnel: [w226 w232] -> w218
              tunnel: w197 -> [w225 w227]
              tunnel: w216 -> [w224 _]
              tunnel: w196 -> [w223 w231]
              tunnel: w189 -> [w222 w228]
              frame "raster", Default {
                n89 = call "push_raster_data_as_CS.vi"("number-of-pixels"=w224, "error in"=w223, "fpga_input_vec"=w222, "FPGA Interface"=w225) -> ("error out"=w226:errorcluster)  [unwired: 6 in, 1 out]
              }
              frame "CS" {
                n90 = call "cast_meta_idx_toFXP.vi"("error in"=w231, "cs-traj-data-in"=w228) -> ("error out"=w230:errorcluster, "cs-traj-data-out"=w229:fxp<+/-,16,5>[])  [unwired: 8 in]
                n91 = call "write_FXP_16-5_data_to_fpga.vi"("error in"=w230, "all rows"=w229, "FPGA Interface"=w227) -> ("error out"=w232:errorcluster)  [unwired: 7 in, 1 out]
              }
            }
            n92 = Increment(x=w194) -> (x+1=w195:i16)
            n93 = Merge Errors(w214, w220, w218) -> (w219:errorcluster)
          }
          frame Error {
          }
        }
        n94 = feedback-in #1(w132) -> ()
        n95 = Bundle By Name(cluster=w125, "status"=w123) -> (w124:errorcluster)
        n96 = Decrement(x=w133) -> (x-1=w139:i32)
        n97 = xnode "Read/Write Control"("FPGA VI Reference In"=w149, "error in"=w125) -> ("FPGA VI Reference Out"=w145:refnum<k20>, "error out"=w144:errorcluster, "scan-status"=w129:T21, "current-state"=w128:u8)
        n98 = case shown="No Error" w124 {
          selector: w124 -> [w169 w188]
          tunnel: w153 -> [w180 _]
          tunnel: w152 -> [w172 _]
          tunnel: [w171 w188] -> w141
          tunnel: w136 -> [w166 _]
          tunnel: w135 -> [w167 _]
          tunnel: w127 -> [w165 _]
          tunnel: [w165 _] -> w126
          frame No Error {
            w173 = 0 ("number_of_lines")
            n99 = local read "state-machine-params"() -> (w175:T2)
            n100 = local read "z_axis_params"() -> (w176:T5)
            n101 = local read "control_data_path"() -> (w164:path)
            n102 = local read "Ki-y"() -> (w174:sgl)
            n103 = shared-variable ".\\fpga_interface.lvlib\\MasterStop.lvlib\\MasterStop"(FALSE ("MasterStop"), error in=w169) -> (error out=w168:errorcluster)
            n104 = Bundle By Name(cluster=T18 {"Ki_xy"=7.0, "number_of_lines"=0, "Ki_derate"=0.01, "ze_sched_thresh"=0.0, "scan_meta"={"npix"=0, "raster_freq"=0.0, "width"=0.0, "points_per_line"=0, "points_per_period"=0, "total_num_points"=0, "scan_type"=enum."raster", "number_of_scans"=0, "actual_sub_samble_perc"=0.0, "mu_length"=0.0, "tip_velocity"=0.0, "pix_idx"=[], "overscan_samples"=0, "pre_scan_samples"=0}, "z_axis_params"={"z_u_max"=5.0, "setpoint_scan"=-0.3000030517578125, "Ki_scan"=0.02, "uz_safe"=0.0, "Kiz_down"=0.02, "setpoint_up"=-0.899993896484375, "do_Dz"=FALSE, "PID_while_xy_move"=FALSE, "TF_params"={"TF_order"=0, "Num"=[0.0, 0.0, 0.0, 0.0, 0.0, 0.0, 0.0, 0.0, 0.0], "Den"=[0.0, 0.0, 0.0, 0.0, 0.0, 0.0, 0.0, 0.0, 0.0]}, "KI_slope"=0.0, "enable_KI_sched"=FALSE, "KI_min"=0.0, "KI_max"=0.0}, "state_counts"=[], "state_machine_params"={"xy_settled_samples_threshold"=0, "xy_error_threshold"=0.01, "zup_err_threshold"=0.0, "prescan_samples"=-12144, "TOL"=256.0, "collect_all"=TRUE, "numEntities"=256}, "input_data_path"=path "", "output_data_path"=path "", "xy_control_path"=path ""} ("raster_asCS__meta_out"), "xy_control_path"=w164, "Ki_xy"=w174, "number_of_lines"=w173, "Ki_derate"=w173, "ze_sched_thresh"=w173, "scan_meta"=w180, "z_axis_params"=w176, "state_counts"=w172, "state_machine_params"=w175, "input_data_path"=w166, "output_data_path"=w165) -> (w177:T18)
            n105 = Open/Create/Replace File(file path (use dialog)=w167, operation (0:open)=T16."replace or create") -> (refnum out=w184:refnum<file>)  [unwired: 4 in, 2 out]
            n106 = call <vilib>:"Flatten To JSON String.vi"("Numeric Extensions (F)"=TRUE, "error in (no error)"=w168, "Variant"=w177) -> ("error out"=w181:errorcluster, "JSON String"=w182:string)  [unwired: 7 in]
            n107 = Write to Binary File(file (use dialog)=w184, data=w182, error in=w181, 5:FALSE ("prepend array or string size? (T)")) -> (refnum out=w185:refnum<file>, error out=w186:errorcluster)  [unwired: 2 in, 1 out]
            n108 = Close File(refnum=w185, error in=w186) -> (error out=w171:errorcluster)  [unwired: 1 out]
          }
          frame Error {
          }
        }
        n109 = Equal?(x=w138, y=w139) -> (x = y?=w148:bool)
        n110 = local write "current-state"(w128) -> ()
        n111 = local write "scan-status"(w129) -> ()
        n112 = Or(x=w148, y=w147) -> (x .or. y?=w146:bool)
        n113 = case shown="False" w146 {
          tunnel: w145 -> [w158 w163]
          tunnel: w144 -> [w156 w162]
          tunnel: [w158 w161] -> w143
          tunnel: [w155 w160] -> w140
          frame False {
            n114 = shared-variable ".\\fpga_interface.lvlib\\Host2fpgaFIFOFilled"(FALSE ("Host2fpgaFIFOFilled"), error in=w156) -> (error out=w155:errorcluster)
            n115 = local write "trigger-0"(TRUE ("trigger-0")) -> ()
          }
          frame True {
            w159 = TRUE ("ABORT")
            n116 = xnode "Read/Write Control"("FPGA VI Reference In"=w163, "error in"=w162, "ABORT"=w159, "stop"=w159) -> ("FPGA VI Reference Out"=w161:refnum<k20>, "error out"=w160:errorcluster)
            n117 = local write "STOP"(w159) -> ()
          }
        }
        n118 = Merge Errors(w140, w141) -> (w142:errorcluster)
        "current-acquisition" <- w133
      }
      "Array 3" <- w79
      "output-data-paths" <- w78
      n119 = xnode "Invoke Method"("FPGA VI Reference In"=w90, "error in"=w91, "IRQ Number(s)"=0, "Timeout (ms)"=5000) -> ("FPGA VI Reference Out"=w98:refnum<k20>, "error out"=w97:errorcluster, "IRQ(s) Asserted"=w99:i32)  [unwired: 1 out]
      n120 = case shown="True" "Alert-on-Finish" {
        tunnel: w91 -> [_ _]
        frame False {
        }
        frame True {
          n121 = call <vilib>:"Beep.vi"("use system alert? (T)"=FALSE, "duration (msec)"=u32 1000, "frequency (Hz)"=u32 400) -> ()  [unwired: 9 in]
        }
      }
      n122 = xnode "Invoke Method"("FPGA VI Reference In"=w98, "error in"=w97, "IRQ Number(s)"=w99) -> ("FPGA VI Reference Out"=w94:refnum<k20>, "error out"=w93:errorcluster)
      n123 = xnode "Close FPGA VI Reference"("FPGA VI Reference In"=w94, "error in"=w93) -> ("error out"=w58:errorcluster)
    }
  }
  "error out" <- w7
